vi "Destroy.vi"(8 "error in (no error)":errorcluster, 11 "Conditional in":refnum<class "Case Structure.lvclass">) -> (0 "error out":errorcluster)   [LabVIEW 2020, in "Test Executive.lvlib" / "Case Structure.lvclass"]
uses:
  <vilib>/gpm_packages/@cs/test-executive/Source/Test Executive/Case Structure/Case Structure.lvclass
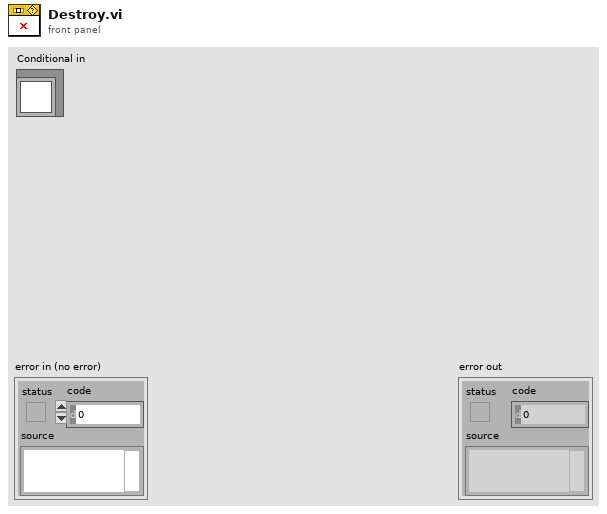
[diagram p1: front panel]
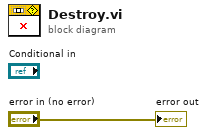
[diagram p0: block diagram]
diagram:
  "error out" <- "error in (no error)"
